vi "pulse_tester_16IQ.vi"() -> ()   [LabVIEW 2021]
uses:
  CTL/emitter params.ctl
  CTL/mode_type.ctl
  pdw.ctl
  <vilib>/measure/maspectr.llb/FFT Power Spectrum and PSD for 1 Chan (CDB).vi
  <vilib>/Analysis/NI_AALPro.lvlib
  <vilib>/measure/NI_MAPro.lvlib
  <instrlib>/_niInstr/Basic Elements/v1/FPGA/niInstr Basic Elements v1 FPGA.lvlib
panel:
  out "D phase to Dt":dbl[](graph)
  out "output valid":i16[](graph)
  in  "tx rate":i32=50
  out "Cluster":T1={"PW"=60000, "frequency shift"=0.004999999999999005, "amp"=0.31623077392578125, "mode type"=enum."LFM", "mode depth"=234562481, "mode filter"=0, "phase shift"=0.0, "pulse shape filter"=0}
  out "Array":i32[](array[numeric])
  out "free DDS":i16[](graph)
  out "Power Spectrum / PSD":cluster{"f0":dbl, "df":dbl, "magnitude":dbl[]}[](graph)
  out "amp out":dbl[](graph)
  out "phase out":dbl[](graph)
  in  "num of sampels for test":i32=65000 format="%.0p"
  out "I data":dbl[](graph)
  in  "emmiter":T3[](array[typedef])=[{"f set"=[1000000.0], "hop rate (Hz)"=6000.0, "d.c."=0.9, "amp (dB)"=-10.0, "mod type"=enum."LFM", "mod depth"=10000000.0, "DOA"=0.0, "t start"=0.0, "t end"=0.0}] {"t end" format="%#_3p"; "t start" format="%#_3p"; "DOA" format="%#_3p"; "mod depth" format="%.0p"}
  out "phase in to DDS":dbl[](graph)
  out "frequncy  in to DDS":dbl[](graph)
  in  "Fs":i32=200000000 format="%.0p"
  # "mode type:\n0- cw\n3-lfm\n4- bpsk\n5-qpsk"
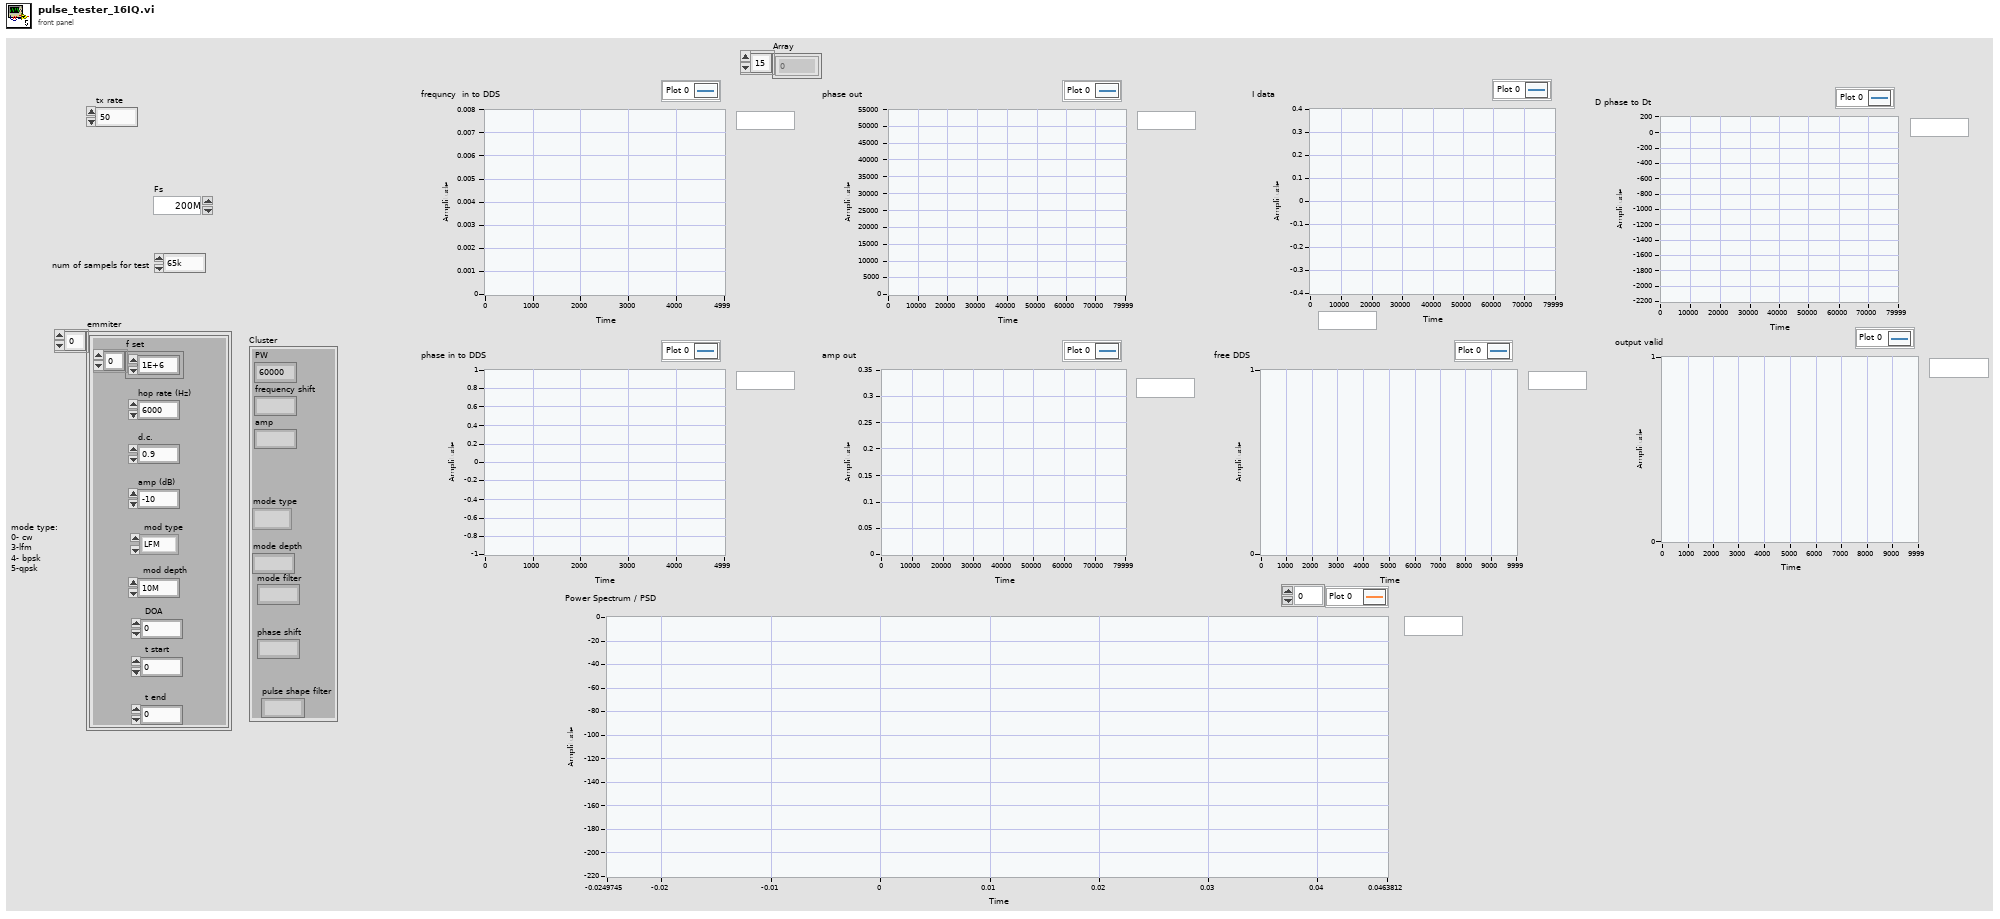
[diagram p1: front panel]
types:
  T1 = typedef "pdw.ctl" = cluster{"PW":u32, "frequency shift":fxp<+/-,48,0>, "amp":fxp<+/-,18,1>, "mode type":T2, "mode depth":u32, "mode filter":u8, "phase shift":fxp<+/-,16,1>, "pulse shape filter":u8}
  T2 = typedef "mode_type.ctl" = enum8{"CW", "NC - CW", "NC - cw", "LFM", "BPSK", "QPSK"}
  T3 = typedef "emitter params.ctl" = cluster{"f set":dbl[], "hop rate (Hz)":dbl, "d.c.":dbl, "amp (dB)":dbl, "mod type":T2, "mod depth":dbl, "DOA":dbl, "t start":dbl, "t end":dbl}
  T4 = typedef "PDW_lv2.ctl" = cluster{"t start":dbl, "frequency (Hz)":dbl, "duration (sec)":dbl, "amp (lin)":dbl, "mod type":T2, "mod depth":dbl, "phase (rad)":dbl[]}
  T5 = typedef "niInstr DSP v1 Shared.lvlib/IQ Data.ctl" = cluster{"I":fxp<+/-,18,1>, "Q":fxp<+/-,18,1>, "overflow":bool}
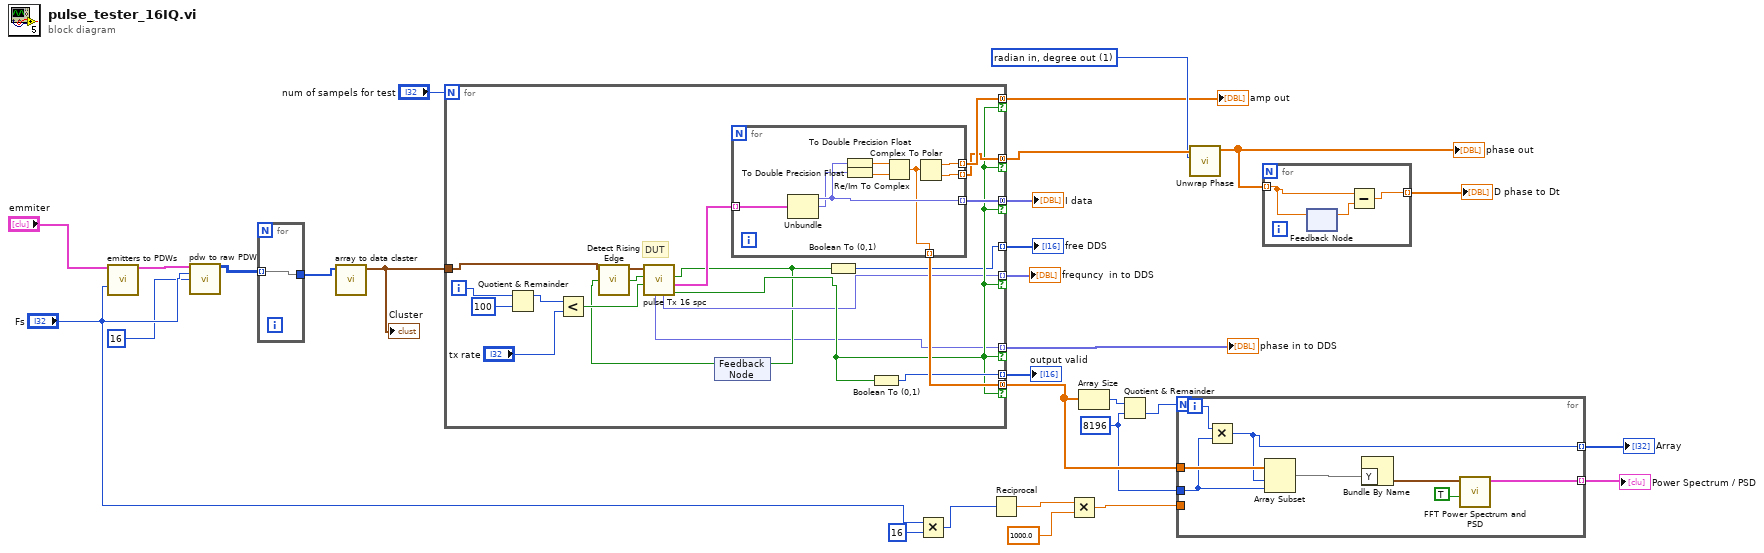
[diagram p0: block diagram]
diagram:
  w16 = 8196 ("length")
  w25 = 1 items=["radian in, radian out", "radian in, degree out", "degree in, degree out", "degree in, radian out"] ("phase unit")
  n1 = call "emitters to PDWs.vi"("emmiter"="emmiter", "center frequency (Hz)"="Fs") -> ("sorted array"=w22:T4[])  [unwired: 11 in, 2 out]
  n2 = call "pdw to raw PDW.vi"("PDWs"=w22, "Fs fpGa"="Fs", "SPC"=16) -> ("Array"=w10:u64[][])  [unwired: 10 in, 2 out]
  n3 = for {
    tunnel: [w30] -> w4
    tunnel: w10 -> [w30] mode=indexing
  }
  n4 = call "array to data claster.vi"("Array"=w4) -> ("Cluster"=w3:T1)  [unwired: 10 in]
  "Cluster" <- w3
  n5 = for {
    N: "num of sampels for test" -> [_]
    tunnel: [w49] -> w29 mode=concatenating if=w35
    tunnel: [w34] -> w28 mode=indexing if=w35
    tunnel: [w31] -> w27 mode=indexing if=w35
    tunnel: [w47] -> w26 mode=concatenating if=w35
    tunnel: [w48] -> w24 mode=concatenating if=w35
    tunnel: [w46] -> w21 mode=concatenating if=w35
    tunnel: [w33] -> w19 mode=indexing
    tunnel: [w40] -> w13 mode=indexing
    tunnel: w3 -> [w36]
    i -> [w45]
    # "DUT"
    n6 = Quotient & Remainder(x=w45, y=100) -> (x-y*floor(x/y)=w43:i32)  [unwired: 1 out]
    n7 = Less?(x=w43, y="tx rate") -> (x < y?=w41:bool)
    n8 = feedback #1() -> (w39:bool)  [unwired: 1 in]
    n9 = call <instrlib>:"Detect Rising Edge.vi"("signal"=w39) -> ("edge detected"=w38:bool)  [unwired: 14 in]
    n10 = call "pulse Tx 16 spc.vi"("enable line"=w41, "take it!"=w38, "Cluster"=w36) -> ("output valid"=w35:bool, "IQ out"=w37:T5[], "free dds"=w32:bool, "frequncy"=w34:fxp<+/-,48,0>, "phase"=w31:fxp<+/-,16,1>)  [unwired: 4 in]
    n11 = feedback-in #1(w32) -> ()
    n12 = for {
      tunnel: w37 -> [w57] mode=indexing
      tunnel: [w56] -> w49 mode=indexing
      tunnel: [w54] -> w48 mode=indexing
      tunnel: [w53] -> w47 mode=indexing
      tunnel: [w52] -> w46 mode=indexing
      n13 = Unbundle(w57) -> ("I"=w56:fxp<+/-,18,1>, "Q"=w55:fxp<+/-,18,1>)  [unwired: 1 out]
      n14 = To Double Precision Float(number=w56) -> (double precision float=w51:dbl)
      n15 = To Double Precision Float(number=w55) -> (double precision float=w50:dbl)
      n16 = Re/Im To Complex(1:w50, 2:w51) -> (0:w52:cdb)
      n17 = Complex To Polar(r * e^(i*theta)=w52) -> (r=w54:dbl, theta=w53:dbl)
    }
    n18 = Boolean To (0,1)(Boolean=w32) -> (0, 1=w33:i16)
    n19 = Boolean To (0,1)(Boolean=w35) -> (0, 1=w40:i16)
  }
  "frequncy  in to DDS" <- w28
  "phase in to DDS" <- w27
  "I data" <- w29
  "amp out" <- w24
  "free DDS" <- w19
  "output valid" <- w13
  n20 = Multiply(x="Fs", y=16) -> (x*y=w8:i32)
  n21 = Reciprocal(x=w8) -> (1/x=w7:dbl)
  n22 = Multiply(x=w7, y=1000.0) -> (x*y=w5:dbl)
  n23 = Array Size(array=w21) -> (size(s)=w17:i32)
  n24 = Quotient & Remainder(x=w17, y=w16) -> (floor(x/y)=w15:i32)  [unwired: 1 out]
  n25 = for {
    N: w15 -> [_]
    tunnel: w21 -> [w62]
    tunnel: w5 -> [_]
    tunnel: w16 -> [w61]
    tunnel: [w59] -> w14 mode=indexing
    tunnel: [w60] -> w18 mode=indexing
    i -> [w58]
    n26 = Multiply(x=w58, y=w61) -> (x*y=w60:i32)
    n27 = Array Subset(array=w62, index=w60, length=w61) -> (w63:cdb[])
    n28 = Bundle By Name("Y"=w63) -> (w65:waveform(cdb))  [unwired: 1 in]
    n29 = call-poly <vilib>:"FFT Power Spectrum and PSD.vi"("dB On (F)"=TRUE, "time signal"=w65) -> ("Power Spectrum / PSD"=w59:cluster{"f0":dbl, "df":dbl, "magnitude":dbl[]})  [unwired: 6 in, 3 out]
  }
  "Power Spectrum / PSD" <- w14
  "Array" <- w18
  n30 = call <vilib>:"Unwrap Phase.vi"("phase unit"=w25, "Phase"=w26) -> ("Unwrapped Phase"=w12:dbl[])  [unwired: 8 in, 1 out]
  "phase out" <- w12
  n31 = for {
    tunnel: w12 -> [w68] mode=indexing
    tunnel: [w66] -> w11 mode=indexing
    n32 = feedback-in #2(w68) -> ()
    n33 = feedback #2() -> (w67:dbl)  [unwired: 1 in]
    n34 = Subtract(x=w68, y=w67) -> (x-y=w66:dbl)
  }
  "D phase to Dt" <- w11
